vi "Initialize Node Resources.vi"(8 "error in":errorcluster) -> (0 "error out":errorcluster, 3 "Communication FIFOs":T1)   [LabVIEW 2014, in "IO Node Logic Template_SPIBus0.lvlib"]
uses:
  IO Node Logic Template_SPIBus0.lvlib
  <vilib>/rvi/LocalResourceManager/LocalResourceManager.xnode
  <vilib>/rvi/DataTransferAndStorage/Container/Common/niFpgaContainerGetUniqueNameForEmu.vi
  <vilib>/rvi/DataTransferAndStorage/Container/Common/niFpgaContainerSetEmuInfo.vi
  <vilib>/rvi/eio/common/nirviEmuReportErrorAndStop.vi
  Node/Controls/NodeResources FIFOs.ctl
  Controls/All Nodes Resources.ctl
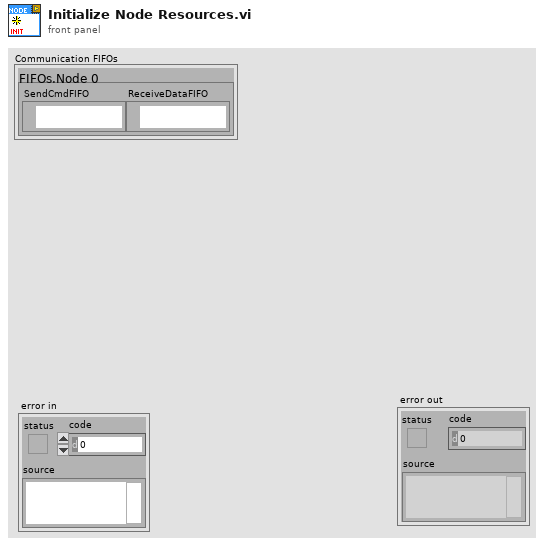
[diagram p1: front panel]
types:
  T1 = typedef "IO Node Logic Template_SPIBus0.lvlib/All Nodes Resources.ctl" = cluster{"FIFOs.Node 0":T2}
  T2 = typedef "IO Node Logic Template_SPIBus0.lvlib/NodeResources FIFOs.ctl" = cluster{"SendCmdFIFO":refnum<k21>, "ReceiveDataFIFO":refnum<k21>}
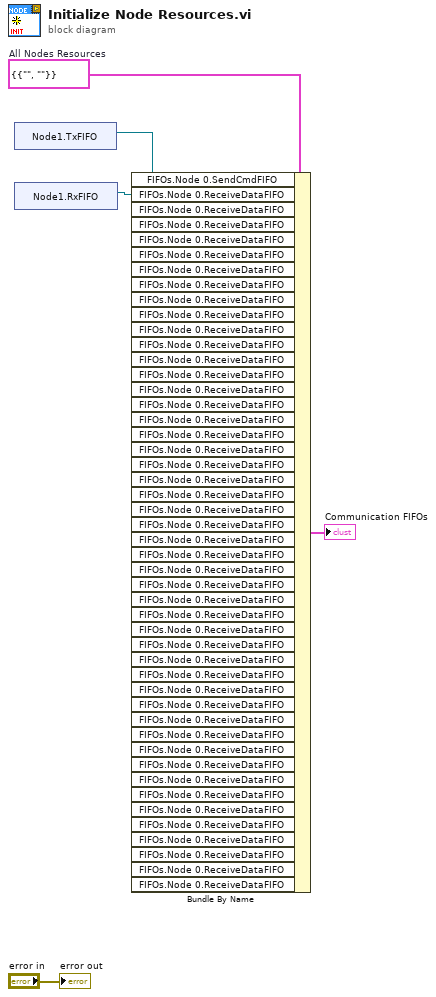
[diagram p0: block diagram]
diagram:
  w5 = T1 {"FIFOs.Node 0"={"SendCmdFIFO"="", "ReceiveDataFIFO"=""}}  # All Nodes Resources
  n1 = xnode "Node1.TxFIFO"() -> ("FIFO Out"=w4:refnum<k21>)
  n2 = xnode "Node1.RxFIFO"() -> ("FIFO Out"=w3:refnum<k21>)
  n3 = Bundle By Name(cluster=w5, "FIFOs.Node 0.SendCmdFIFO"=w4, "FIFOs.Node 0.ReceiveDataFIFO"=w3) -> (→"Communication FIFOs":T1)  [unwired: 46 in]
  "error out" <- "error in"
